vi "Draw.vi"(8 "error in (no error)":errorcluster, 11 "Text in":refnum<class "Text.lvclass">) -> (0 "error out":errorcluster, 2 "Picture":picture, 3 "Text out":refnum<class "Text.lvclass">)   [LabVIEW 2017, in "LV Image Editor Framework.lvlib" / "Text.lvclass"]
uses:
  Text.lvclass
  C:/Github/LIEF/Forms/Shape/Shape.lvclass
  Shape/Shape.lvclass/Shape.ctl
  Text.lvclass/Text.ctl
  Shape/Shape.lvclass
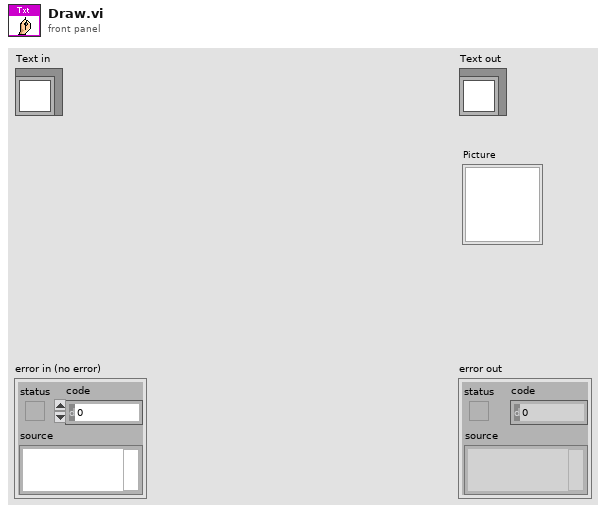
[diagram p1: front panel]
types:
  T1 = enum16{"User-specified Font", "Application Font", "System Font", "Dialog Font"}
  T2 = cluster{"Font Name:":string, "Size":i16, "Strikeout?":bool, "Italic?":bool, "Underline?":bool, "Outline?":bool, "Shadow?":bool, "Bold?":bool}
  T3 = cluster{"Left":i32, "Top":i32, "Right":i32, "Bottom":i32}
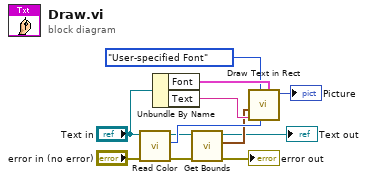
[diagram p0: block diagram]
diagram:
  n1 = call "Read Color.vi"("error in (no error)"="error in (no error)", "Shape in"="Text in") -> ("error out"=w5:errorcluster, "Color"=w10:u32, "Shape out"=w3:refnum<class "Text.lvclass">)  [unwired: 7 in]
  n2 = Unbundle By Name("Text in") -> ("Font"=w11:T2, "Text"=w12:string)
  n3 = call "Get Bounds.vi"("error in (no error)"=w5, "Shape in"=w3) -> ("error out"=→"error out":errorcluster, "Bounds"=w9:T3, "Shape out"=→"Text out":refnum<class "Text.lvclass">)  [unwired: 7 in]
  n4 = call <vilib>:"Draw Text in Rect.vi"("[user-specified font]"=w11, "text color(black)"=w10, "desired font(Application)"=T1."User-specified Font", "text"=w12, "rect"=w9) -> ("new picture"=→"Picture":picture)  [unwired: 6 in]
